vi "Initialize pulse counter.vi"(11 "Samples per channel":i32) -> (0 "error out":errorcluster, 3 "DAQmx Task Name":refnum<k21>)   [LabVIEW 2012]
uses:
  Channels.vi
  <vilib>/DAQmx/create/channels.llb/DAQmx Create Channel (CI-Count Edges).vi
  <vilib>/DAQmx/configure/timing.llb/DAQmx Timing (Sample Clock).vi
  <resource>/objmgr/daqmx.rc
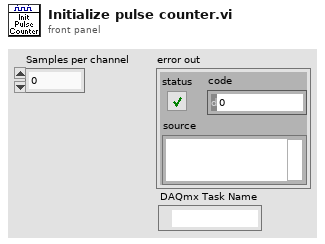
[diagram p1: front panel]
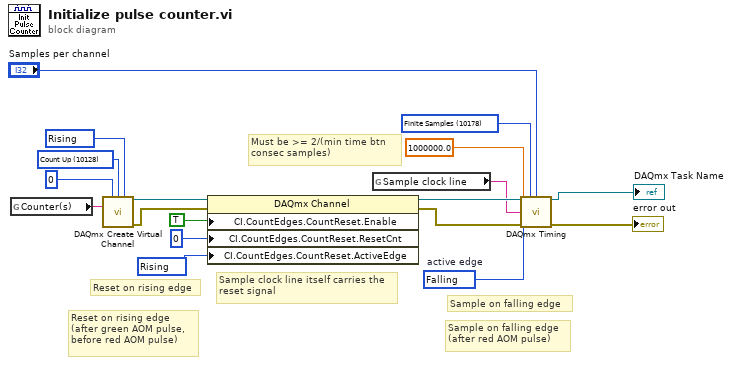
[diagram p0: block diagram]
diagram:
  w10 = 10280 items=["Rising"=10280, "Falling"=10171] ("Edge")
  w9 = 10128 items=["Count Up"=10128, "Count Down"=10124, "Externally Controlled"=10326] ("Count Direction")
  w6 = 10280 items=["Rising"=10280, "Falling"=10171] ("Reset Edge")
  w11 = 10178 items=["Finite Samples"=10178, "Continuous Samples"=10123] ("sample mode")
  w7 = 10171 items=["Rising"=10280, "Falling"=10171]  # active edge
  # "Sample on falling edge\n(after red AOM pulse)"
  # "Reset on rising edge\n(after green AOM pulse,\nbefore red AOM pulse)"
  # "Must be >= 2/(min time btn\nconsec samples)"
  # "Sample on falling edge"
  # "Reset on rising edge"
  # "Sample clock line itself carries the\nreset signal"
  n1 = global read "Channels.vi" "Counter(s)"() -> (w5:tag)
  n2 = call-poly <vilib>:"DAQmx Create Virtual Channel.vi"("initial count"=u32 0 ("Initial Count"), "count direction"=w9, "edge"=w10, "counter"=w5) -> ("task out"=w15:refnum<k21>, "error out"=w18:errorcluster)  [unwired: 10 in]
  n3 = property class="DAQmx Channel"(reference=w15, error in=w18, "CI.CountEdges.CountReset.Enable"=TRUE, "CI.CountEdges.CountReset.ResetCnt"=u32 0 ("Reset Count"), "CI.CountEdges.CountReset.ActiveEdge"=w6) -> (reference out=w16:refnum<k21>, error out=w17:errorcluster)
  n4 = global read "Channels.vi" "Sample clock line"() -> (w4:tag)
  n5 = call-poly <vilib>:"DAQmx Timing.vi"("task/channels in"=w16, "sample mode"=w11, "samples per channel"="Samples per channel", "rate"=1000000.0 ("Rate"), "source"=w4, "active edge"=w7, "error in"=w17) -> ("task out"=→"DAQmx Task Name":refnum<k21>, "error out"=→"error out":errorcluster)  [unwired: 7 in]
